vi "ExtractLogTokens.vi"(0 "HTML":string, 1 "section":string) -> (2 "Before":string, 3 "tagged text":string, 4 "After":string)   [LabVIEW 2012]
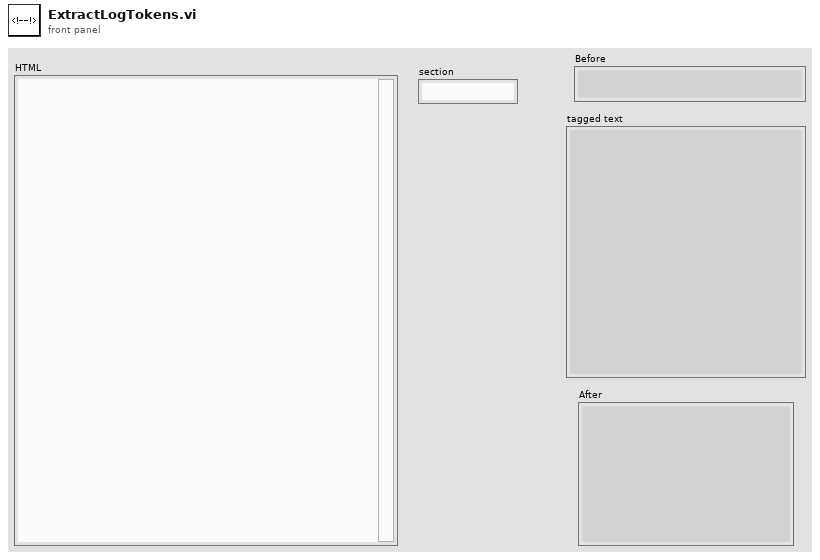
[diagram p1: front panel]
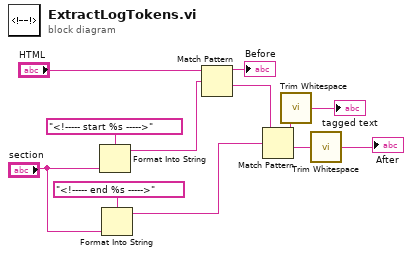
[diagram p0: block diagram]
diagram:
  n1 = Format Into String(format string="<!----- start %s ----->", "section") -> (resulting string=w9:string)  [unwired: 2 in, 1 out]
  n2 = Format Into String(format string="<!----- end %s ----->", "section") -> (resulting string=w5:string)  [unwired: 2 in, 1 out]
  n3 = Match Pattern(string="HTML", regular expression=w9) -> (before substring=→"Before":string, after substring=w8:string)  [unwired: 1 in, 2 out]
  n4 = Match Pattern(string=w8, regular expression=w5) -> (before substring=w3:string, after substring=w4:string)  [unwired: 1 in, 2 out]
  n5 = call <vilib>:"Trim Whitespace.vi"("string"=w3) -> ("trimmed string"=→"tagged text":string)  [unwired: 1 in]
  n6 = call <vilib>:"Trim Whitespace.vi"("string"=w4) -> ("trimmed string"=→"After":string)  [unwired: 1 in]
